vi "Create Ackermann Frame.vi"(8 "error in (no error)":errorcluster) -> (0 "error out":errorcluster, 3 "ackermann steering frame out":refnum<class "NI_Robotics_Ackermann Steering Frame.lvclass">)   [LabVIEW 2012]
uses:
  <vilib>/robotics/Steering/Ackermann Steering Frame/NI_Robotics_Ackermann Steering Frame.lvclass
  <vilib>/robotics/Steering/Ackermann Steering Frame/Ackermann Wheel Group.ctl
  <vilib>/robotics/Steering/Steering Wheel/NI_Robotics_Steering Wheel.lvclass
  <vilib>/robotics/Steering/Fixed Wheel/NI_Robotics_Fixed Wheel.lvclass
  <vilib>/robotics/Steering/Wheel/Wheel Parameters.ctl
  <vilib>/robotics/Steering/Wheel/Rotation Direction.ctl
  <vilib>/robotics/Steering/Steering Wheel/Steering Wheel Parameters.ctl
  <vilib>/robotics/Steering/Steering Wheel/Steering Angle Range.ctl
  <vilib>/robotics/Steering/Steering Wheel/Create Steering Wheel.vi
  <vilib>/robotics/Steering/Fixed Wheel/Create Fixed Wheel.vi
  <vilib>/robotics/Steering/Ackermann Steering Frame/Create Ackermann Steering Frame.vi
  <vilib>/robotics/Steering/Steering Frame/NI_Robotics_Steering Frame.lvclass
  <vilib>/robotics/Steering/Wheel/NI_Robotics_Wheel.lvclass
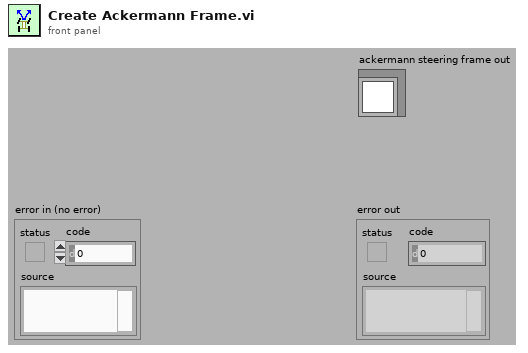
[diagram p1: front panel]
types:
  T1 = typedef "NI_Robotics_Ackermann Steering Frame.lvclass/Ackermann Wheel Group.ctl" = cluster{"Front Left Wheel":refnum<class "NI_Robotics_Steering Wheel.lvclass">, "Front Right Wheel":refnum<class "NI_Robotics_Steering Wheel.lvclass">, "Rear Left Wheel":refnum<class "NI_Robotics_Fixed Wheel.lvclass">, "Rear Right Wheel":refnum<class "NI_Robotics_Fixed Wheel.lvclass">}
  T2 = typedef "NI_Robotics_Wheel.lvclass/Wheel Parameters.ctl" = cluster{"wheel radius":dbl, "gear ratio":dbl, "forward rotation direction":T3}
  T3 = typedef "NI_Robotics_Wheel.lvclass/Rotation Direction.ctl" = u16
  T4 = typedef "NI_Robotics_Steering Wheel.lvclass/Steering Wheel Parameters.ctl" = cluster{"steering gear ratio":dbl, "motor angle offset (rad)":dbl, "steering angle range":T5}
  T5 = typedef "NI_Robotics_Steering Wheel.lvclass/Steering Angle Range.ctl" = cluster{"min steering angle (rad)":dbl, "max steering angle (rad)":dbl}
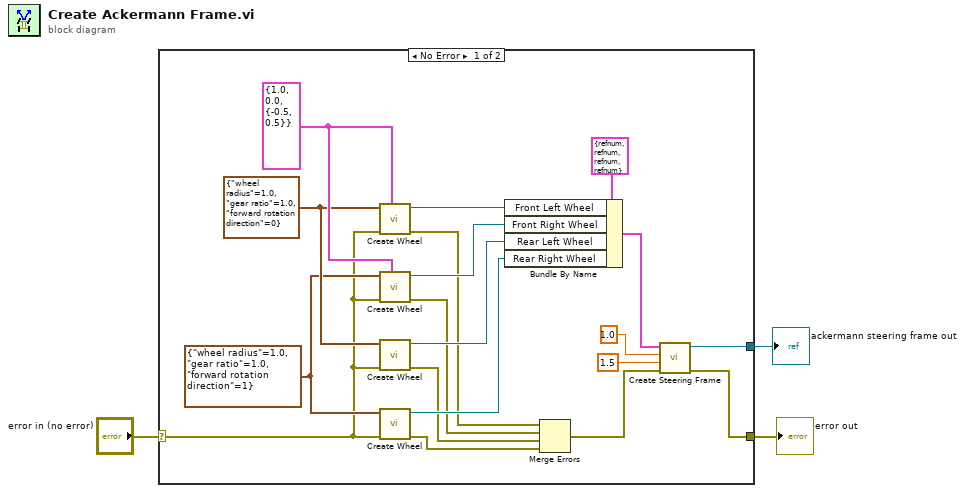
[diagram p0: block diagram]
diagram:
  n1 = case shown="No Error" "error in (no error)" {
    selector: "error in (no error)" -> [w4 w23]
    tunnel: [w16 _] -> w3
    tunnel: [w14 w23] -> w2
    frame No Error {
      w11 = T2 {"wheel radius"=1.0, "gear ratio"=1.0, "forward rotation direction"=1} ("wheel parameters")
      w13 = T4 {"steering gear ratio"=1.0, "motor angle offset (rad)"=0.0, "steering angle range"={"min steering angle (rad)"=-0.5, "max steering angle (rad)"=0.5}} ("steering parameters")
      w12 = T2 {"wheel radius"=1.0, "gear ratio"=1.0, "forward rotation direction"=0} ("wheel parameters")
      n2 = call-poly <vilib>:"Create Wheel.vi"("steering parameters"=w13, "error in (no error)"=w4, "wheel parameters"=w12) -> ("error out"=w5:errorcluster, "steering wheel out"=w22:refnum<class "NI_Robotics_Steering Wheel.lvclass">)  [unwired: 7 in]
      n3 = call-poly <vilib>:"Create Wheel.vi"("steering parameters"=w13, "error in (no error)"=w4, "wheel parameters"=w11) -> ("error out"=w6:errorcluster, "steering wheel out"=w21:refnum<class "NI_Robotics_Steering Wheel.lvclass">)  [unwired: 7 in]
      n4 = call-poly <vilib>:"Create Wheel.vi"("error in (no error)"=w4, "wheel parameters"=w12) -> ("error out"=w7:errorcluster, "fixed wheel out"=w20:refnum<class "NI_Robotics_Fixed Wheel.lvclass">)  [unwired: 8 in]
      n5 = call-poly <vilib>:"Create Wheel.vi"("error in (no error)"=w4, "wheel parameters"=w11) -> ("error out"=w8:errorcluster, "fixed wheel out"=w19:refnum<class "NI_Robotics_Fixed Wheel.lvclass">)  [unwired: 8 in]
      n6 = Bundle By Name(cluster=T1 {"Front Left Wheel"=refnum, "Front Right Wheel"=refnum, "Rear Left Wheel"=refnum, "Rear Right Wheel"=refnum} ("wheels"), "Front Left Wheel"=w22, "Front Right Wheel"=w21, "Rear Left Wheel"=w20, "Rear Right Wheel"=w19) -> (w17:T1)
      n7 = Merge Errors(w5, w6, w7, w8) -> (w15:errorcluster)
      n8 = call-poly <vilib>:"Create Steering Frame.vi"("error in (no error)"=w15, "wheel separation length"=1.5, "wheel separation width"=1.0, "wheels"=w17) -> ("error out"=w14:errorcluster, "ackermann steering frame out"=w16:refnum<class "NI_Robotics_Ackermann Steering Frame.lvclass">)  [unwired: 6 in]
    }
    frame Error {
    }
  }
  "ackermann steering frame out" <- w3
  "error out" <- w2
